vi "InclinometerTest.vi"() -> ()   [LabVIEW 2016]
uses:
  Telemetry/TelemetryFields.ctl
  <vilib>/rvi/DataTransferAndStorage/Container/XNode/niFpgaContainer.xnode
  <vilib>/rvi/FIFO/Fifo_Resource/nirvififoEmulationWrite.vi
  <vilib>/rvi/FIFO/Fifo_Resource/nirvififoEmulationRead.vi
  Inclinometer/InclinometerErrorCodes.ctl
panel:
  out "ZenithAngle":sgl
  out "ErrorCodeTimestamp":u64
  out "ErrorCode":T1
  out "SampleTimestamp":u64
  out "RxFrames":u64
  out "TxFrames":u64
  out "RxBytes":u64
  out "TxBytes":u64
  out "RawAngle":u32
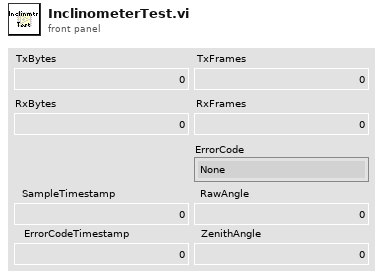
[diagram p1: front panel]
types:
  T1 = typedef "InclinometerErrorCodes.ctl" = enum8{"None", "ResponseAddressError", "ResponseFunctionCodeError", "ResponseByteCountError", "ResponseCRCError", "ResponseUnknownError", "ResponseTimeoutError", "SensorReportsIllegalFunction", "SensorReportsIllegalDataAddress"}
  T2 = cluster{"Timestamp":u64, "TxBytes":u64, "RxBytes":u64, "TxFrames":u64, "RxFrames":u64, "ErrorCode":enum16{"None", "ResponseUnknownError", "ResponseInvalidError", "ResponseTimeoutError", "SensorIndicatesInvalidCommandError", "SensorIndicatesCommunicationTimeoutError", "SensorIndicatesDataLengthError", "SensorIndicatesNumberOfParametersError", "SensorIndicatesParameterError", "SensorIndicatesCommunicationError", "SensorIndicatesIDNumberError", "SensorIndicatesExpansionLineError", "SensorIndicatesWriteControlError"}}
  T3 = cluster{"Timestamp":u64, "TxBytes":u64, "RxBytes":u64, "TxFrames":u64, "RxFrames":u64, "Sensor1Raw":i32, "Sensor2Raw":i32, "Sensor3Raw":i32, "Sensor4Raw":i32, "Sensor5Raw":i32, "Sensor6Raw":i32, "Sensor7Raw":i32, "Sensor8Raw":i32, "Sensor1Eng":sgl, "Sensor2Eng":sgl, "Sensor3Eng":sgl, "Sensor4Eng":sgl, "Sensor5Eng":sgl, "Sensor6Eng":sgl, "Sensor7Eng":sgl, "Sensor8Eng":sgl, "PositionX":sgl, "PositionY":sgl, "PositionZ":sgl, "RotationX":sgl, "RotationY":sgl, "RotationZ":sgl}
  T4 = typedef "TelemetryFields.ctl" = enum16{"None", "InclinometerTxBytes", "InclinometerRxBytes", "InclinometerTxFrames", "InclinometerRxFrames", "InclinometerErrorTimestamp", "InclinometerErrorCode", "InclinometerSampleTimestamp", "InclinometerRawAngle", "InclinometerZenithAngle", "DisplacementTxBytes", "DisplacementRxBytes", "DisplacementTxFrames", "DisplacementRxFrames", "DisplacementErrorTimestamp", "DisplacementErrorCode", "DisplacementSampleTimestamp", "DisplacementRaw1", "DisplacementRaw2", "DisplacementRaw3", "DisplacementRaw4", "DisplacementRaw5", "DisplacementRaw6", "DisplacementRaw7", "DisplacementRaw8", "DisplacementEng1", "DisplacementEng2", "DisplacementEng3", "DisplacementEng4", "DisplacementEng5", "DisplacementEng6", "DisplacementEng7", "DisplacementEng8", "DisplacementPositionX", "DisplacementPositionY", "DisplacementPositionZ", "DisplacementRotationX", "DisplacementRotationY", "DisplacementRotationZ", "AccelerometerSampleCount", "AccelerometerSampleTimestamp", "AccelerometerRaw1", "AccelerometerRaw2", "AccelerometerRaw3", "AccelerometerRaw4", "AccelerometerRaw5", "AccelerometerRaw6", "AccelerometerRaw7", "AccelerometerRaw8", "AccelerometerEng1", "AccelerometerEng2", "AccelerometerEng3", "AccelerometerEng4", "AccelerometerEng5", "AccelerometerEng6", "AccelerometerEng7", "AccelerometerEng8", "AngularAccelerationX", "AngularAccelerationY", "AngularAccelerationZ", "GyroTxBytes", "GyroRxBytes", "GyroTxFrames", "GyroRxFrames", "GyroErrorTimestamp", "GyroErrorCode", "GyroSampleTimestamp", "AngularVelocityX", "AngularVelocityY", "AngularVelocityZ", "GyroStatus", "GyroSequenceNumber", "GyroTemperature", "GyroBITTimestamp", "GyroBIT0", "GyroBIT1", "GyroBIT2", "GyroBIT3", "GyroBIT4", "GyroBIT5", "GyroBIT6", "GyroBIT7"}
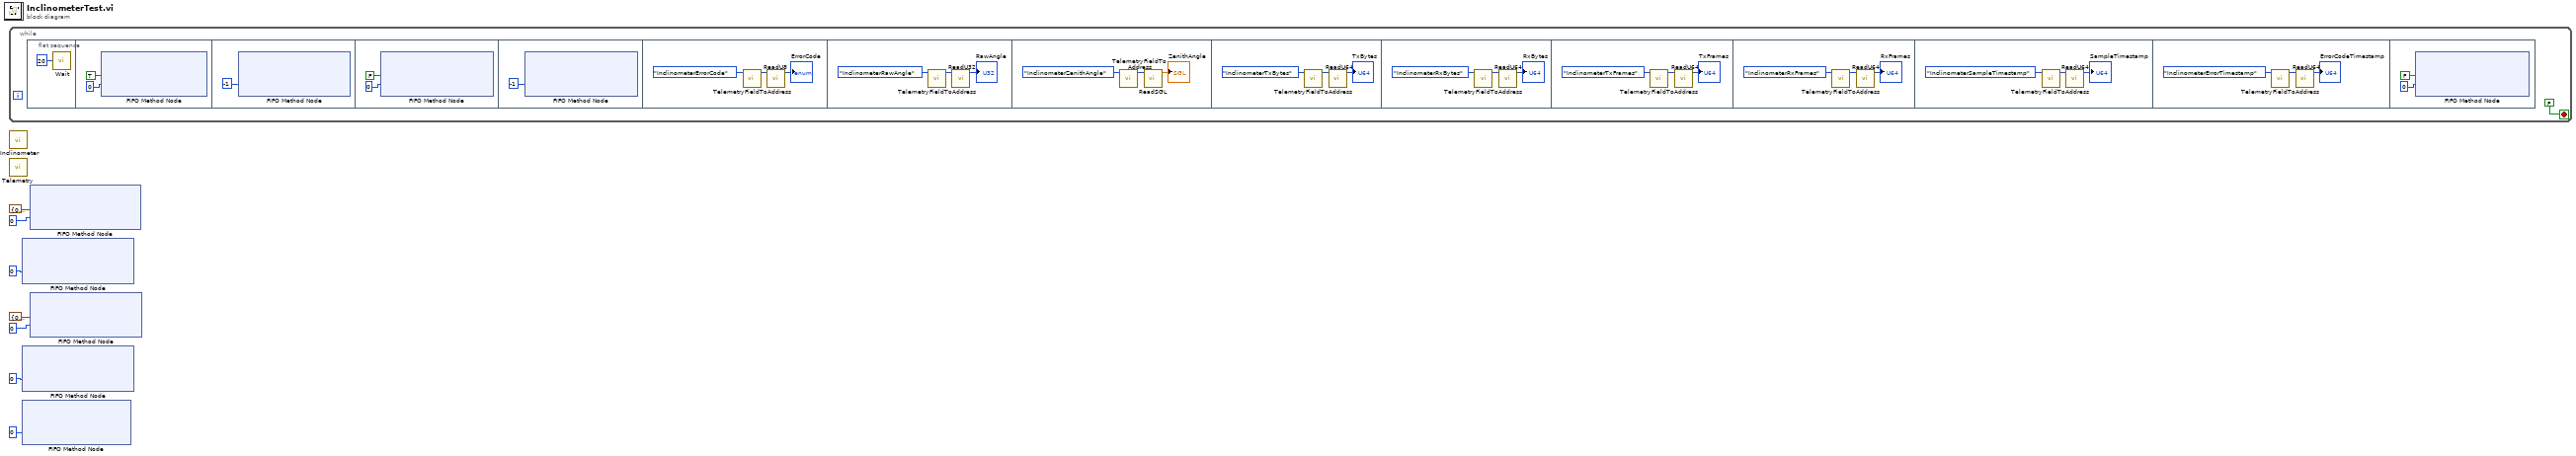
[diagram p0: block diagram]
diagram:
  n1 = while {
    stop <- FALSE stop-if-true
    n2 = flat-sequence {
      frame #0 {
        n3 = call "Wait"("Count(mSec)"=u32 20) -> ()  [unwired: 1 out]
      }
      frame #1 {
        n4 = xnode ("FIFO Method Node")("Element"=TRUE, "Timeout"=0) -> ()  [unwired: 1 in, 2 out]
      }
      frame #2 {
        n5 = xnode ("FIFO Method Node")("Timeout"=-1) -> ()  [unwired: 1 in, 3 out]
      }
      frame #3 {
        n6 = xnode ("FIFO Method Node")("Element"=FALSE, "Timeout"=0) -> ()  [unwired: 1 in, 2 out]
      }
      frame #4 {
        n7 = xnode ("FIFO Method Node")("Timeout"=-1) -> ()  [unwired: 1 in, 3 out]
      }
      frame #5 {
        n8 = call "TelemetryFieldToAddress.vi"("TelemetryFields"=TelemetryFields."InclinometerErrorCode") -> ("Address"=w18:u32)  [unwired: 10 in]
        n9 = call "ReadU8.vi"("Address"=w18) -> ("Data"=→"ErrorCode":u8)  [unwired: 10 in]
      }
      frame #6 {
        n10 = call "TelemetryFieldToAddress.vi"("TelemetryFields"=TelemetryFields."InclinometerRawAngle") -> ("Address"=w20:u32)  [unwired: 10 in]
        n11 = call "ReadU32.vi"("Address"=w20) -> ("Data"=→"RawAngle":u32)  [unwired: 10 in]
      }
      frame #7 {
        n12 = call "TelemetryFieldToAddress.vi"("TelemetryFields"=TelemetryFields."InclinometerZenithAngle") -> ("Address"=w23:u32)  [unwired: 10 in]
        n13 = call "ReadSGL.vi"("Address"=w23) -> ("Data"=→"ZenithAngle":sgl)  [unwired: 10 in]
      }
      frame #8 {
        n14 = call "TelemetryFieldToAddress.vi"("TelemetryFields"=TelemetryFields."InclinometerTxBytes") -> ("Address"=w26:u32)  [unwired: 10 in]
        n15 = call "ReadU64.vi"("Address"=w26) -> ("Data"=→"TxBytes":u64)  [unwired: 10 in]
      }
      frame #9 {
        n16 = call "TelemetryFieldToAddress.vi"("TelemetryFields"=TelemetryFields."InclinometerRxBytes") -> ("Address"=w29:u32)  [unwired: 10 in]
        n17 = call "ReadU64.vi"("Address"=w29) -> ("Data"=→"RxBytes":u64)  [unwired: 10 in]
      }
      frame #10 {
        n18 = call "TelemetryFieldToAddress.vi"("TelemetryFields"=TelemetryFields."InclinometerTxFrames") -> ("Address"=w32:u32)  [unwired: 10 in]
        n19 = call "ReadU64.vi"("Address"=w32) -> ("Data"=→"TxFrames":u64)  [unwired: 10 in]
      }
      frame #11 {
        n20 = call "TelemetryFieldToAddress.vi"("TelemetryFields"=TelemetryFields."InclinometerRxFrames") -> ("Address"=w35:u32)  [unwired: 10 in]
        n21 = call "ReadU64.vi"("Address"=w35) -> ("Data"=→"RxFrames":u64)  [unwired: 10 in]
      }
      frame #12 {
        n22 = call "TelemetryFieldToAddress.vi"("TelemetryFields"=TelemetryFields."InclinometerSampleTimestamp") -> ("Address"=w38:u32)  [unwired: 10 in]
        n23 = call "ReadU64.vi"("Address"=w38) -> ("Data"=→"SampleTimestamp":u64)  [unwired: 10 in]
      }
      frame #13 {
        n24 = call "TelemetryFieldToAddress.vi"("TelemetryFields"=TelemetryFields."InclinometerErrorTimestamp") -> ("Address"=w41:u32)  [unwired: 10 in]
        n25 = call "ReadU64.vi"("Address"=w41) -> ("Data"=→"ErrorCodeTimestamp":u64)  [unwired: 10 in]
      }
      frame #14 {
        n26 = xnode ("FIFO Method Node")("Element"=FALSE, "Timeout"=0) -> ()  [unwired: 1 in, 2 out]
      }
    }
  }
  n27 = call "Inclinometer.vi"() -> ()  [unwired: 12 in]
  n28 = call "Telemetry.vi"() -> ()  [unwired: 12 in]
  n29 = xnode ("FIFO Method Node")("Timeout"=0) -> ()  [unwired: 1 in, 3 out]
  n30 = xnode ("FIFO Method Node")("Timeout"=0) -> ()  [unwired: 1 in, 3 out]
  n31 = xnode ("FIFO Method Node")("Timeout"=0) -> ()  [unwired: 1 in, 3 out]
  n32 = xnode ("FIFO Method Node")("Element"=T3 {"Timestamp"=0, "TxBytes"=0, "RxBytes"=0, "TxFrames"=0, "RxFrames"=0, "Sensor1Raw"=0, "Sensor2Raw"=0, "Sensor3Raw"=0, "Sensor4Raw"=0, "Sensor5Raw"=0, "Sensor6Raw"=0, "Sensor7Raw"=0, "Sensor8Raw"=0, "Sensor1Eng"=0.0, "Sensor2Eng"=0.0, "Sensor3Eng"=0.0, "Sensor4Eng"=0.0, "Sensor5Eng"=0.0, "Sensor6Eng"=0.0, "Sensor7Eng"=0.0, "Sensor8Eng"=0.0, "PositionX"=0.0, "PositionY"=0.0, "PositionZ"=0.0, "RotationX"=0.0, "RotationY"=0.0, "RotationZ"=0.0}, "Timeout"=0) -> ()  [unwired: 1 in, 2 out]
  n33 = xnode ("FIFO Method Node")("Element"=T2 {"Timestamp"=0, "TxBytes"=0, "RxBytes"=0, "TxFrames"=0, "RxFrames"=0, "ErrorCode"=enum."None"}, "Timeout"=0) -> ()  [unwired: 1 in, 2 out]
